vi "Temperature Control Main.vi"(8 "error in (no error)":errorcluster) -> (0 "error out":errorcluster)   [LabVIEW 2014]
uses:
  state machine.ctl
panel:
  in  "Stop Button":bool
  out "status":string
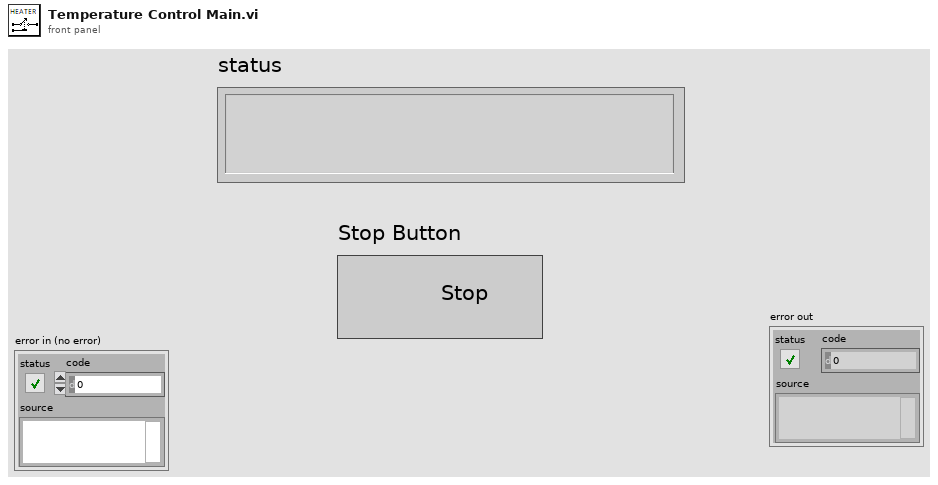
[diagram p1: front panel]
types:
  T1 = typedef "state machine.ctl" = enum16{"Init", "Wait For Main Power", "Main Power ON", "Compare Temperature", "Turn ON Heater", "Turn OFF Heater", "Error Handling", "Shutdown"}
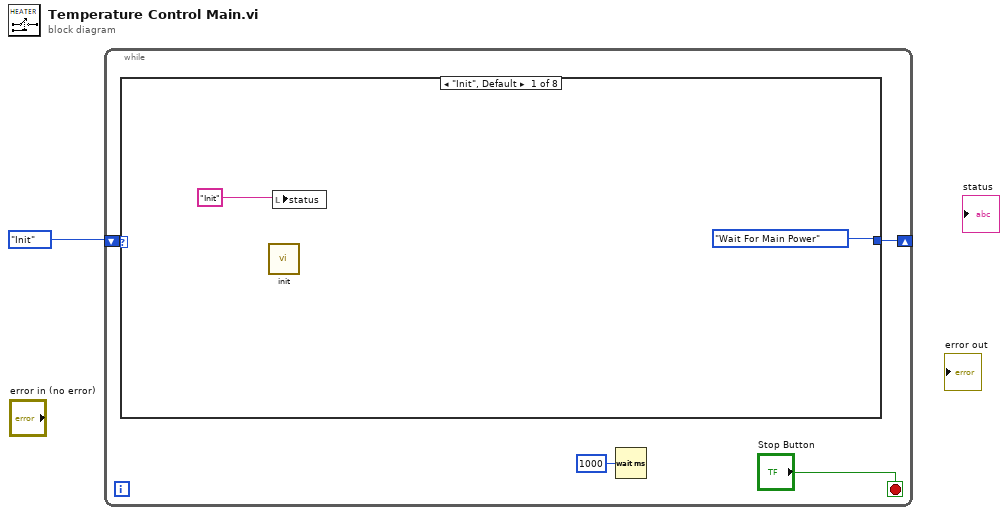
[diagram p0: block diagram]
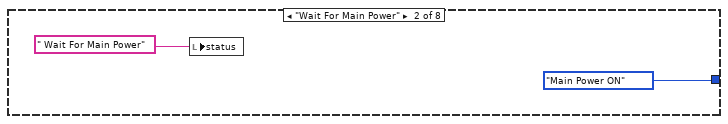
[diagram p2: hidden frame]
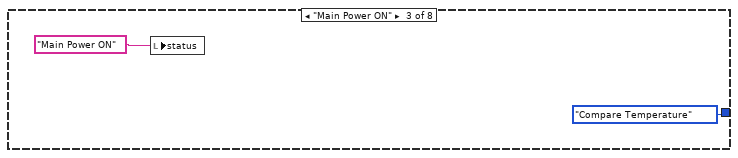
[diagram p3: hidden frame]
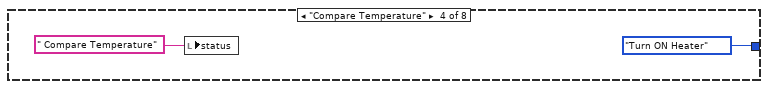
[diagram p4: hidden frame]
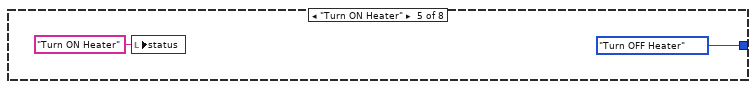
[diagram p5: hidden frame]
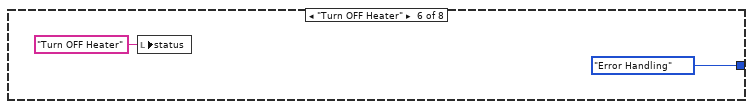
[diagram p6: hidden frame]
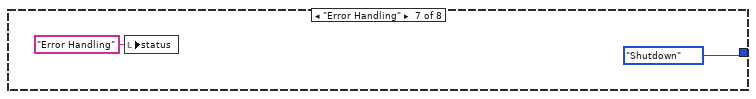
[diagram p7: hidden frame]
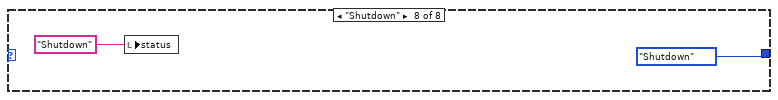
[diagram p8: hidden frame]
diagram:
  n1 = while {
    shift-right: [w3] -> _
    shift-left: state_machine."Init" ("state") -> [w4]
    stop <- "Stop Button" stop-if-true
    n2 = case shown="\"Init\", Default" w4 {
      tunnel: [state_machine."Wait For Main Power" ("state") state_machine."Main Power ON" ("state") state_machine."Compare Temperature" ("state") state_machine."Turn ON Heater" ("state") state_machine."Turn OFF Heater" ("state") state_machine."Error Handling" ("state") state_machine."Shutdown" ("state") state_machine."Shutdown" ("state")] -> w3
      frame "Init", Default {
        n3 = call "init.vi"() -> ()  [unwired: 4 in, 2 out]
        n4 = local write "status"("Init") -> ()
      }
      frame "Wait For Main Power" {
        n5 = local write "status"(" Wait For Main Power" ("user display")) -> ()
      }
      frame "Main Power ON" {
        n6 = local write "status"("Main Power ON" ("user display")) -> ()
      }
      frame "Compare Temperature" {
        n7 = local write "status"(" Compare Temperature" ("status")) -> ()
      }
      frame "Turn ON Heater" {
        n8 = local write "status"("Turn ON Heater" ("status")) -> ()
      }
      frame "Turn OFF Heater" {
        n9 = local write "status"("Turn OFF Heater" ("status")) -> ()
      }
      frame "Error Handling" {
        n10 = local write "status"("Error Handling" ("status")) -> ()
      }
      frame "Shutdown" {
        n11 = local write "status"("Shutdown" ("status")) -> ()
      }
    }
    n12 = Wait (ms)(milliseconds to wait=u32 1000) -> ()  [unwired: 1 out]
  }
